vi "App - analyze RUS V6.vi"() -> ()   [LabVIEW 2018] (continued)
  in  "t.folder file path array":T26[](array[typedef])=[{"temperature"=241.719, "temperature str"="241.71900", "file path"=path "D:/Data/Ultrasound/LSCO/LSCO22__130814c/5_Cooling_2nd_try/September_2014/091614/241.71900K_500_2500_2.10000V_0.00000T_Sep16-2014__11-57-01_001_091614.bin", "last mod"=timestamp(3493727821 s since 1904-01-01), "file name str"="D:\\Data\\Ultrasound\\LSCO\\LSCO22__130814c\\5_Cooling_2nd_try\\September_2014\\091614\\241.71900K_500_2500_2.10000V_0.00000T_Sep16-2014__11-57-01_001_091614.bin", "mod time(min)"=58228797.016666666, "file format"=enum."binary", "power(V)"=2.1, "Magn Field(T) "=0.0}, {"temperature"=220.002, "temperature str"="220.00200", "file path"=path "D:/Data/Ultrasound/LSCO/LSCO22__130814c/5_Cooling_2nd_try/September_2014/091614/220.00200K_500_2500_2.10000V_0.00000T_Sep16-2014__12-18-19_001_091614.bin", "last mod"=timestamp(3493729099 s since 1904-01-01), "file name str"="D:\\Data\\Ultrasound\\LSCO\\LSCO22__130814c\\5_Cooling_2nd_try\\September_2014\\091614\\220.00200K_500_2500_2.10000V_0.00000T_Sep16-2014__12-18-19_001_091614.bin", "mod time(min)"=58228818.31666667, "file format"=enum."binary", "power(V)"=2.1, "Magn Field(T) "=0.0}, {"temperature"=219.999, "temperature str"="219.99900", "file path"=path "D:/Data/Ultrasound/LSCO/LSCO22__130814c/5_Cooling_2nd_try/September_2014/091614/219.99900K_500_2500_2.10000V_0.00000T_Sep16-2014__12-20-36_001_091614.bin", "last mod"=timestamp(3493729236 s since 1904-01-01), "file name str"="D:\\Data\\Ultrasound\\LSCO\\LSCO22__130814c\\5_Cooling_2nd_try\\September_2014\\091614\\219.99900K_500_2500_2.10000V_0.00000T_Sep16-2014__12-20-36_001_091614.bin", "mod time(min)"=58228820.6, "file format"=enum."binary", "power(V)"=2.1, "Magn Field(T) "=0.0}, {"temperature"=220.002, "temperature str"="220.00200", "file path"=path "D:/Data/Ultrasound/LSCO/LSCO22__130814c/5_Cooling_2nd_try/September_2014/091614/220.00200K_500_2500_2.10000V_0.00000T_Sep16-2014__12-21-56_001_091614.bin", "last mod"=timestamp(3493729316 s since 1904-01-01), "file name str"="D:\\Data\\Ultrasound\\LSCO\\LSCO22__130814c\\5_Cooling_2nd_try\\September_2014\\091614\\220.00200K_500_2500_2.10000V_0.00000T_Sep16-2014__12-21-56_001_091614.bin", "mod time(min)"=58228821.93333333, "file format"=enum."binary", "power(V)"=2.1, "Magn Field(T) "=0.0}, {"temperature"=221.376, "temperature str"="221.37600", "file path"=path "D:/Data/Ultrasound/LSCO/LSCO22__130814c/5_Cooling_2nd_try/September_2014/091614/221.37600K_500_2500_2.10000V_0.00000T_Sep16-2014__12-23-15_001_091614.bin", "last mod"=timestamp(3493729395 s since 1904-01-01), "file name str"="D:\\Data\\Ultrasound\\LSCO\\LSCO22__130814c\\5_Cooling_2nd_try\\September_2014\\091614\\221.37600K_500_2500_2.10000V_0.00000T_Sep16-2014__12-23-15_001_091614.bin", "mod time(min)"=58228823.25, "file format"=enum."binary", "power(V)"=2.1, "Magn Field(T) "=0.0}, {"temperature"=220.736, "temperature str"="220.73600", "file path"=path "D:/Data/Ultrasound/LSCO/LSCO22__130814c/5_Cooling_2nd_try/September_2014/091614/220.73600K_500_2500_2.10000V_0.00000T_Sep16-2014__12-24-35_001_091614.bin", "last mod"=timestamp(3493729475 s since 1904-01-01), "file name str"="D:\\Data\\Ultrasound\\LSCO\\LSCO22__130814c\\5_Cooling_2nd_try\\September_2014\\091614\\220.73600K_500_2500_2.10000V_0.00000T_Sep16-2014__12-24-35_001_091614.bin", "mod time(min)"=58228824.583333336, "file format"=enum."binary", "power(V)"=2.1, "Magn Field(T) "=0.0}, {"temperature"=220.112, "temperature str"="220.11200", "file path"=path "D:/Data/Ultrasound/LSCO/LSCO22__130814c/5_Cooling_2nd_try/September_2014/091614/220.11200K_500_2500_2.10000V_0.00000T_Sep16-2014__12-25-54_001_091614.bin", "last mod"=timestamp(3493729554 s since 1904-01-01), "file name str"="D:\\Data\\Ultrasound\\LSCO\\LSCO22__130814c\\5_Cooling_2nd_try\\September_2014\\091614\\220.11200K_500_2500_2.10000V_0.00000T_Sep16-2014__12-25-54_001_091614.bin", "mod time(min)"=58228825.9, "file format"=enum."binary", "power(V)"=2.1, "Magn Field(T) "=0.0}, {"temperature"=219.885, "temperature str"="219.88500", "file path"=path "D:/Data/Ultrasound/LSCO/LSCO22__130814c/5_Cooling_2nd_try/September_2014/091614/219.88500K_500_2500_2.10000V_0.00000T_Sep16-2014__12-27-13_001_091614.bin", "last mod"=timestamp(3493729633 s since 1904-01-01), "file name str"="D:\\Data\\Ultrasound\\LSCO\\LSCO22__130814c\\5_Cooling_2nd_try\\September_2014\\091614\\219.88500K_500_2500_2.10000V_0.00000T_Sep16-2014__12-27-13_001_091614.bin", "mod time(min)"=58228827.21666667, "file format"=enum."binary", "power(V)"=2.1, "Magn Field(T) "=0.0}, {"temperature"=219.907, "temperature str"="219.90700", "file path"=path "D:/Data/Ultrasound/LSCO/LSCO22__130814c/5_Cooling_2nd_try/September_2014/091614/219.90700K_500_2500_2.10000V_0.00000T_Sep16-2014__12-28-33_001_091614.bin", "last mod"=timestamp(3493729713 s since 1904-01-01), "file name str"="D:\\Data\\Ultrasound\\LSCO\\LSCO22__130814c\\5_Cooling_2nd_try\\September_2014\\091614\\219.90700K_500_2500_2.10000V_0.00000T_Sep16-2014__12-28-33_001_091614.bin", "mod time(min)"=58228828.55, "file format"=enum."binary", "power(V)"=2.1, "Magn Field(T) "=0.0}, {"temperature"=220.061, "temperature str"="220.06100", "file path"=path "D:/Data/Ultrasound/LSCO/LSCO22__130814c/5_Cooling_2nd_try/September_2014/091614/220.06100K_500_2500_2.10000V_0.00000T_Sep16-2014__12-29-52_001_091614.bin", "last mod"=timestamp(3493729792 s since 1904-01-01), "file name str"="D:\\Data\\Ultrasound\\LSCO\\LSCO22__130814c\\5_Cooling_2nd_try\\September_2014\\091614\\220.06100K_500_2500_2.10000V_0.00000T_Sep16-2014__12-29-52_001_091614.bin", "mod time(min)"=58228829.86666667, "file format"=enum."binary", "power(V)"=2.1, "Magn Field(T) "=0.0}, {"temperature"=220.167, "temperature str"="220.16700", "file path"=path "D:/Data/Ultrasound/LSCO/LSCO22__130814c/5_Cooling_2nd_try/September_2014/091614/220.16700K_500_2500_2.10000V_0.00000T_Sep16-2014__12-31-11_001_091614.bin", "last mod"=timestamp(3493729871 s since 1904-01-01), "file name str"="D:\\Data\\Ultrasound\\LSCO\\LSCO22__130814c\\5_Cooling_2nd_try\\September_2014\\091614\\220.16700K_500_2500_2.10000V_0.00000T_Sep16-2014__12-31-11_001_091614.bin", "mod time(min)"=58228831.18333333, "file format"=enum."binary", "power(V)"=2.1, "Magn Field(T) "=0.0}, {"temperature"=220.232, "temperature str"="220.23200", "file path"=path "D:/Data/Ultrasound/LSCO/LSCO22__130814c/5_Cooling_2nd_try/September_2014/091614/220.23200K_500_2500_2.10000V_0.00000T_Sep16-2014__12-32-31_001_091614.bin", "last mod"=timestamp(3493729951 s since 1904-01-01), "file name str"="D:\\Data\\Ultrasound\\LSCO\\LSCO22__130814c\\5_Cooling_2nd_try\\September_2014\\091614\\220.23200K_500_2500_2.10000V_0.00000T_Sep16-2014__12-32-31_001_091614.bin", "mod time(min)"=58228832.516666666, "file format"=enum."binary", "power(V)"=2.1, "Magn Field(T) "=0.0}, {"temperature"=220.32, "temperature str"="220.32000", "file path"=path "D:/Data/Ultrasound/LSCO/LSCO22__130814c/5_Cooling_2nd_try/September_2014/091614/220.32000K_500_2500_2.10000V_0.00000T_Sep16-2014__12-33-50_001_091614.bin", "last mod"=timestamp(3493730030 s since 1904-01-01), "file name str"="D:\\Data\\Ultrasound\\LSCO\\LSCO22__130814c\\5_Cooling_2nd_try\\September_2014\\091614\\220.32000K_500_2500_2.10000V_0.00000T_Sep16-2014__12-33-50_001_091614.bin", "mod time(min)"=58228833.833333336, "file format"=enum."binary", "power(V)"=2.1, "Magn Field(T) "=0.0}, {"temperature"=220.447, "temperature str"="220.44700", "file path"=path "D:/Data/Ultrasound/LSCO/LSCO22__130814c/5_Cooling_2nd_try/September_2014/091614/220.44700K_500_2500_2.10000V_0.00000T_Sep16-2014__12-35-10_001_091614.bin", "last mod"=timestamp(3493730110 s since 1904-01-01), "file name str"="D:\\Data\\Ultrasound\\LSCO\\LSCO22__130814c\\5_Cooling_2nd_try\\September_2014\\091614\\220.44700K_500_2500_2.10000V_0.00000T_Sep16-2014__12-35-10_001_091614.bin", "mod time(min)"=58228835.166666664, "file format"=enum."binary", "power(V)"=2.1, "Magn Field(T) "=0.0}, {"temperature"=220.033, "temperature str"="220.03300", "file path"=path "D:/Data/Ultrasound/LSCO/LSCO22__130814c/5_Cooling_2nd_try/September_2014/091614/220.03300K_500_2500_2.10000V_0.00000T_Sep16-2014__12-36-29_001_091614.bin", "last mod"=timestamp(3493730189 s since 1904-01-01), "file name str"="D:\\Data\\Ultrasound\\LSCO\\LSCO22__130814c\\5_Cooling_2nd_try\\September_2014\\091614\\220.03300K_500_2500_2.10000V_0.00000T_Sep16-2014__12-36-29_001_091614.bin", "mod time(min)"=58228836.483333334, "file format"=enum."binary", "power(V)"=2.1, "Magn Field(T) "=0.0}, {"temperature"=219.225, "temperature str"="219.22500", "file path"=path "D:/Data/Ultrasound/LSCO/LSCO22__130814c/5_Cooling_2nd_try/September_2014/091614/219.22500K_500_2500_2.10000V_0.00000T_Sep16-2014__12-37-48_001_091614.bin", "last mod"=timestamp(3493730268 s since 1904-01-01), "file name str"="D:\\Data\\Ultrasound\\LSCO\\LSCO22__130814c\\5_Cooling_2nd_try\\September_2014\\091614\\219.22500K_500_2500_2.10000V_0.00000T_Sep16-2014__12-37-48_001_091614.bin", "mod time(min)"=58228837.8, "file format"=enum."binary", "power(V)"=2.1, "Magn Field(T) "=0.0}, {"temperature"=219.76, "temperature str"="219.76000", "file path"=path "D:/Data/Ultrasound/LSCO/LSCO22__130814c/5_Cooling_2nd_try/September_2014/091614/219.76000K_500_2500_2.10000V_0.00000T_Sep16-2014__12-39-08_001_091614.bin", "last mod"=timestamp(3493730348 s since 1904-01-01), "file name str"="D:\\Data\\Ultrasound\\LSCO\\LSCO22__130814c\\5_Cooling_2nd_try\\September_2014\\091614\\219.76000K_500_2500_2.10000V_0.00000T_Sep16-2014__12-39-08_001_091614.bin", "mod time(min)"=58228839.13333333, "file format"=enum."binary", "power(V)"=2.1, "Magn Field(T) "=0.0}, {"temperature"=220.195, "temperature str"="220.19500", "file path"=path "D:/Data/Ultrasound/LSCO/LSCO22__130814c/5_Cooling_2nd_try/September_2014/091614/220.19500K_500_2500_2.10000V_0.00000T_Sep16-2014__12-40-27_001_091614.bin", "last mod"=timestamp(3493730427 s since 1904-01-01), "file name str"="D:\\Data\\Ultrasound\\LSCO\\LSCO22__130814c\\5_Cooling_2nd_try\\September_2014\\091614\\220.19500K_500_2500_2.10000V_0.00000T_Sep16-2014__12-40-27_001_091614.bin", "mod time(min)"=58228840.45, "file format"=enum."binary", "power(V)"=2.1, "Magn Field(T) "=0.0}, {"temperature"=219.549, "temperature str"="219.54900", "file path"=path "D:/Data/Ultrasound/LSCO/LSCO22__130814c/5_Cooling_2nd_try/September_2014/091614/219.54900K_500_2500_2.10000V_0.00000T_Sep16-2014__12-41-46_001_091614.bin", "last mod"=timestamp(3493730506 s since 1904-01-01), "file name str"="D:\\Data\\Ultrasound\\LSCO\\LSCO22__130814c\\5_Cooling_2nd_try\\September_2014\\091614\\219.54900K_500_2500_2.10000V_0.00000T_Sep16-2014__12-41-46_001_091614.bin", "mod time(min)"=58228841.766666666, "file format"=enum."binary", "power(V)"=2.1, "Magn Field(T) "=0.0}, {"temperature"=219.085, "temperature str"="219.08500", "file path"=path "D:/Data/Ultrasound/LSCO/LSCO22__130814c/5_Cooling_2nd_try/September_2014/091614/219.08500K_500_2500_2.10000V_0.00000T_Sep16-2014__12-43-06_001_091614.bin", "last mod"=timestamp(3493730586 s since 1904-01-01), "file name str"="D:\\Data\\Ultrasound\\LSCO\\LSCO22__130814c\\5_Cooling_2nd_try\\September_2014\\091614\\219.08500K_500_2500_2.10000V_0.00000T_Sep16-2014__12-43-06_001_091614.bin", "mod time(min)"=58228843.1, "file format"=enum."binary", "power(V)"=2.1, "Magn Field(T) "=0.0}, {"temperature"=219.006, "temperature str"="219.00600", "file path"=path "D:/Data/Ultrasound/LSCO/LSCO22__130814c/5_Cooling_2nd_try/September_2014/091614/219.00600K_500_2500_2.10000V_0.00000T_Sep16-2014__12-44-25_001_091614.bin", "last mod"=timestamp(3493730665 s since 1904-01-01), "file name str"="D:\\Data\\Ultrasound\\LSCO\\LSCO22__130814c\\5_Cooling_2nd_try\\September_2014\\091614\\219.00600K_500_2500_2.10000V_0.00000T_Sep16-2014__12-44-25_001_091614.bin", "mod time(min)"=58228844.416666664, "file format"=enum."binary", "power(V)"=2.1, "Magn Field(T) "=0.0}, {"temperature"=218.791, "temperature str"="218.79100", "file path"=path "D:/Data/Ultrasound/LSCO/LSCO22__130814c/5_Cooling_2nd_try/September_2014/091614/218.79100K_500_2500_2.10000V_0.00000T_Sep16-2014__12-45-45_001_091614.bin", "last mod"=timestamp(3493730745 s since 1904-01-01), "file name str"="D:\\Data\\Ultrasound\\LSCO\\LSCO22__130814c\\5_Cooling_2nd_try\\September_2014\\091614\\218.79100K_500_2500_2.10000V_0.00000T_Sep16-2014__12-45-45_001_091614.bin", "mod time(min)"=58228845.75, "file format"=enum."binary", "power(V)"=2.1, "Magn Field(T) "=0.0}, {"temperature"=218.445, "temperature str"="218.44500", "file path"=path "D:/Data/Ultrasound/LSCO/LSCO22__130814c/5_Cooling_2nd_try/September_2014/091614/218.44500K_500_2500_2.10000V_0.00000T_Sep16-2014__12-47-04_001_091614.bin", "last mod"=timestamp(3493730824 s since 1904-01-01), "file name str"="D:\\Data\\Ultrasound\\LSCO\\LSCO22__130814c\\5_Cooling_2nd_try\\September_2014\\091614\\218.44500K_500_2500_2.10000V_0.00000T_Sep16-2014__12-47-04_001_091614.bin", "mod time(min)"=58228847.06666667, "file format"=enum."binary", "power(V)"=2.1, "Magn Field(T) "=0.0}, {"temperature"=218.177, "temperature str"="218.17700", "file path"=path "D:/Data/Ultrasound/LSCO/LSCO22__130814c/5_Cooling_2nd_try/September_2014/091614/218.17700K_500_2500_2.10000V_0.00000T_Sep16-2014__12-48-23_001_091614.bin", "last mod"=timestamp(3493730903 s since 1904-01-01), "file name str"="D:\\Data\\Ultrasound\\LSCO\\LSCO22__130814c\\5_Cooling_2nd_try\\September_2014\\091614\\218.17700K_500_2500_2.10000V_0.00000T_Sep16-2014__12-48-23_001_091614.bin", "mod time(min)"=58228848.38333333, "file format"=enum."binary", "power(V)"=2.1, "Magn Field(T) "=0.0}, {"temperature"=217.946, "temperature str"="217.94600", "file path"=path "D:/Data/Ultrasound/LSCO/LSCO22__130814c/5_Cooling_2nd_try/September_2014/091614/217.94600K_500_2500_2.10000V_0.00000T_Sep16-2014__12-49-43_001_091614.bin", "last mod"=timestamp(3493730983 s since 1904-01-01), "file name str"="D:\\Data\\Ultrasound\\LSCO\\LSCO22__130814c\\5_Cooling_2nd_try\\September_2014\\091614\\217.94600K_500_2500_2.10000V_0.00000T_Sep16-2014__12-49-43_001_091614.bin", "mod time(min)"=58228849.71666667, "file format"=enum."binary", "power(V)"=2.1, "Magn Field(T) "=0.0}, {"temperature"=217.689, "temperature str"="217.68900", "file path"=path "D:/Data/Ultrasound/LSCO/LSCO22__130814c/5_Cooling_2nd_try/September_2014/091614/217.68900K_500_2500_2.10000V_0.00000T_Sep16-2014__12-51-02_001_091614.bin", "last mod"=timestamp(3493731062 s since 1904-01-01), "file name str"="D:\\Data\\Ultrasound\\LSCO\\LSCO22__130814c\\5_Cooling_2nd_try\\September_2014\\091614\\217.68900K_500_2500_2.10000V_0.00000T_Sep16-2014__12-51-02_001_091614.bin", "mod time(min)"=58228851.03333333, "file format"=enum."binary", "power(V)"=2.1, "Magn Field(T) "=0.0}, {"temperature"=217.41, "temperature str"="217.41000", "file path"=path "D:/Data/Ultrasound/LSCO/LSCO22__130814c/5_Cooling_2nd_try/September_2014/091614/217.41000K_500_2500_2.10000V_0.00000T_Sep16-2014__12-52-21_001_091614.bin", "last mod"=timestamp(3493731141 s since 1904-01-01), "file name str"="D:\\Data\\Ultrasound\\LSCO\\LSCO22__130814c\\5_Cooling_2nd_try\\September_2014\\091614\\217.41000K_500_2500_2.10000V_0.00000T_Sep16-2014__12-52-21_001_091614.bin", "mod time(min)"=58228852.35, "file format"=enum."binary", "power(V)"=2.1, "Magn Field(T) "=0.0}, {"temperature"=217.145, "temperature str"="217.14500", "file path"=path "D:/Data/Ultrasound/LSCO/LSCO22__130814c/5_Cooling_2nd_try/September_2014/091614/217.14500K_500_2500_2.10000V_0.00000T_Sep16-2014__12-53-41_001_091614.bin", "last mod"=timestamp(3493731221 s since 1904-01-01), "file name str"="D:\\Data\\Ultrasound\\LSCO\\LSCO22__130814c\\5_Cooling_2nd_try\\September_2014\\091614\\217.14500K_500_2500_2.10000V_0.00000T_Sep16-2014__12-53-41_001_091614.bin", "mod time(min)"=58228853.68333333, "file format"=enum."binary", "power(V)"=2.1, "Magn Field(T) "=0.0}, {"temperature"=216.895, "temperature str"="216.89500", "file path"=path "D:/Data/Ultrasound/LSCO/LSCO22__130814c/5_Cooling_2nd_try/September_2014/091614/216.89500K_500_2500_2.10000V_0.00000T_Sep16-2014__12-55-00_001_091614.bin", "last mod"=timestamp(3493731300 s since 1904-01-01), "file name str"="D:\\Data\\Ultrasound\\LSCO\\LSCO22__130814c\\5_Cooling_2nd_try\\September_2014\\091614\\216.89500K_500_2500_2.10000V_0.00000T_Sep16-2014__12-55-00_001_091614.bin", "mod time(min)"=58228855.0, "file format"=enum."binary", "power(V)"=2.1, "Magn Field(T) "=0.0}, {"temperature"=216.629, "temperature str"="216.62900", "file path"=path "D:/Data/Ultrasound/LSCO/LSCO22__130814c/5_Cooling_2nd_try/September_2014/091614/216.62900K_500_2500_2.10000V_0.00000T_Sep16-2014__12-56-20_001_091614.bin", "last mod"=timestamp(3493731380 s since 1904-01-01), "file name str"="D:\\Data\\Ultrasound\\LSCO\\LSCO22__130814c\\5_Cooling_2nd_try\\September_2014\\091614\\216.62900K_500_2500_2.10000V_0.00000T_Sep16-2014__12-56-20_001_091614.bin", "mod time(min)"=58228856.333333336, "file format"=enum."binary", "power(V)"=2.1, "Magn Field(T) "=0.0}, {"temperature"=216.359, "temperature str"="216.35900", "file path"=path "D:/Data/Ultrasound/LSCO/LSCO22__130814c/5_Cooling_2nd_try/September_2014/091614/216.35900K_500_2500_2.10000V_0.00000T_Sep16-2014__12-57-39_001_091614.bin", "last mod"=timestamp(3493731459 s since 1904-01-01), "file name str"="D:\\Data\\Ultrasound\\LSCO\\LSCO22__130814c\\5_Cooling_2nd_try\\September_2014\\091614\\216.35900K_500_2500_2.10000V_0.00000T_Sep16-2014__12-57-39_001_091614.bin", "mod time(min)"=58228857.65, "file format"=enum."binary", "power(V)"=2.1, "Magn Field(T) "=0.0}, {"temperature"=216.106, "temperature str"="216.10600", "file path"=path "D:/Data/Ultrasound/LSCO/LSCO22__130814c/5_Cooling_2nd_try/September_2014/091614/216.10600K_500_2500_2.10000V_0.00000T_Sep16-2014__12-58-58_001_091614.bin", "last mod"=timestamp(3493731538 s since 1904-01-01), "file name str"="D:\\Data\\Ultrasound\\LSCO\\LSCO22__130814c\\5_Cooling_2nd_try\\September_2014\\091614\\216.10600K_500_2500_2.10000V_0.00000T_Sep16-2014__12-58-58_001_091614.bin", "mod time(min)"=58228858.96666667, "file format"=enum."binary", "power(V)"=2.1, "Magn Field(T) "=0.0}, {"temperature"=215.839, "temperature str"="215.83900", "file path"=path "D:/Data/Ultrasound/LSCO/LSCO22__130814c/5_Cooling_2nd_try/September_2014/091614/215.83900K_500_2500_2.10000V_0.00000T_Sep16-2014__13-00-18_001_091614.bin", "last mod"=timestamp(3493731618 s since 1904-01-01), "file name str"="D:\\Data\\Ultrasound\\LSCO\\LSCO22__130814c\\5_Cooling_2nd_try\\September_2014\\091614\\215.83900K_500_2500_2.10000V_0.00000T_Sep16-2014__13-00-18_001_091614.bin", "mod time(min)"=58228860.3, "file format"=enum."binary", "power(V)"=2.1, "Magn Field(T) "=0.0}, {"temperature"=215.585, "temperature str"="215.58500", "file path"=path "D:/Data/Ultrasound/LSCO/LSCO22__130814c/5_Cooling_2nd_try/September_2014/091614/215.58500K_500_2500_2.10000V_0.00000T_Sep16-2014__13-01-37_001_091614.bin", "last mod"=timestamp(3493731697 s since 1904-01-01), "file name str"="D:\\Data\\Ultrasound\\LSCO\\LSCO22__130814c\\5_Cooling_2nd_try\\September_2014\\091614\\215.58500K_500_2500_2.10000V_0.00000T_Sep16-2014__13-01-37_001_091614.bin", "mod time(min)"=58228861.61666667, "file format"=enum."binary", "power(V)"=2.1, "Magn Field(T) "=0.0}, {"temperature"=215.319, "temperature str"="215.31900", "file path"=path "D:/Data/Ultrasound/LSCO/LSCO22__130814c/5_Cooling_2nd_try/September_2014/091614/215.31900K_500_2500_2.10000V_0.00000T_Sep16-2014__13-02-56_001_091614.bin", "last mod"=timestamp(3493731776 s since 1904-01-01), "file name str"="D:\\Data\\Ultrasound\\LSCO\\LSCO22__130814c\\5_Cooling_2nd_try\\September_2014\\091614\\215.31900K_500_2500_2.10000V_0.00000T_Sep16-2014__13-02-56_001_091614.bin", "mod time(min)"=58228862.93333333, "file format"=enum."binary", "power(V)"=2.1, "Magn Field(T) "=0.0}, {"temperature"=215.053, "temperature str"="215.05300", "file path"=path "D:/Data/Ultrasound/LSCO/LSCO22__130814c/5_Cooling_2nd_try/September_2014/091614/215.05300K_500_2500_2.10000V_0.00000T_Sep16-2014__13-04-16_001_091614.bin", "last mod"=timestamp(3493731856 s since 1904-01-01), "file name str"="D:\\Data\\Ultrasound\\LSCO\\LSCO22__130814c\\5_Cooling_2nd_try\\September_2014\\091614\\215.05300K_500_2500_2.10000V_0.00000T_Sep16-2014__13-04-16_001_091614.bin", "mod time(min)"=58228864.266666666, "file format"=enum."binary", "power(V)"=2.1, "Magn Field(T) "=0.0}, {"temperature"=214.797, "temperature str"="214.79700", "file path"=path "D:/Data/Ultrasound/LSCO/LSCO22__130814c/5_Cooling_2nd_try/September_2014/091614/214.79700K_500_2500_2.10000V_0.00000T_Sep16-2014__13-05-35_001_091614.bin", "last mod"=timestamp(3493731935 s since 1904-01-01), "file name str"="D:\\Data\\Ultrasound\\LSCO\\LSCO22__130814c\\5_Cooling_2nd_try\\September_2014\\091614\\214.79700K_500_2500_2.10000V_0.00000T_Sep16-2014__13-05-35_001_091614.bin", "mod time(min)"=58228865.583333336, "file format"=enum."binary", "power(V)"=2.1, "Magn Field(T) "=0.0}, {"temperature"=214.531, "temperature str"="214.53100", "file path"=path "D:/Data/Ultrasound/LSCO/LSCO22__130814c/5_Cooling_2nd_try/September_2014/091614/214.53100K_500_2500_2.10000V_0.00000T_Sep16-2014__13-06-55_001_091614.bin", "last mod"=timestamp(3493732015 s since 1904-01-01), "file name str"="D:\\Data\\Ultrasound\\LSCO\\LSCO22__130814c\\5_Cooling_2nd_try\\September_2014\\091614\\214.53100K_500_2500_2.10000V_0.00000T_Sep16-2014__13-06-55_001_091614.bin", "mod time(min)"=58228866.916666664, "file format"=enum."binary", "power(V)"=2.1, "Magn Field(T) "=0.0}, {"temperature"=214.276, "temperature str"="214.27600", "file path"=path "D:/Data/Ultrasound/LSCO/LSCO22__130814c/5_Cooling_2nd_try/September_2014/091614/214.27600K_500_2500_2.10000V_0.00000T_Sep16-2014__13-08-14_001_091614.bin", "last mod"=timestamp(3493732094 s since 1904-01-01), "file name str"="D:\\Data\\Ultrasound\\LSCO\\LSCO22__130814c\\5_Cooling_2nd_try\\September_2014\\091614\\214.27600K_500_2500_2.10000V_0.00000T_Sep16-2014__13-08-14_001_091614.bin", "mod time(min)"=58228868.233333334, "file format"=enum."binary", "power(V)"=2.1, "Magn Field(T) "=0.0}, {"temperature"=214.01, "temperature str"="214.01000", "file path"=path "D:/Data/Ultrasound/LSCO/LSCO22__130814c/5_Cooling_2nd_try/September_2014/091614/214.01000K_500_2500_2.10000V_0.00000T_Sep16-2014__13-09-33_001_091614.bin", "last mod"=timestamp(3493732173 s since 1904-01-01), "file name str"="D:\\Data\\Ultrasound\\LSCO\\LSCO22__130814c\\5_Cooling_2nd_try\\September_2014\\091614\\214.01000K_500_2500_2.10000V_0.00000T_Sep16-2014__13-09-33_001_091614.bin", "mod time(min)"=58228869.55, "file format"=enum."binary", "power(V)"=2.1, "Magn Field(T) "=0.0}, {"temperature"=213.745, "temperature str"="213.74500", "file path"=path "D:/Data/Ultrasound/LSCO/LSCO22__130814c/5_Cooling_2nd_try/September_2014/091614/213.74500K_500_2500_2.10000V_0.00000T_Sep16-2014__13-10-53_001_091614.bin", "last mod"=timestamp(3493732253 s since 1904-01-01), "file name str"="D:\\Data\\Ultrasound\\LSCO\\LSCO22__130814c\\5_Cooling_2nd_try\\September_2014\\091614\\213.74500K_500_2500_2.10000V_0.00000T_Sep16-2014__13-10-53_001_091614.bin", "mod time(min)"=58228870.88333333, "file format"=enum."binary", "power(V)"=2.1, "Magn Field(T) "=0.0}, {"temperature"=213.49, "temperature str"="213.49000", "file path"=path "D:/Data/Ultrasound/LSCO/LSCO22__130814c/5_Cooling_2nd_try/September_2014/091614/213.49000K_500_2500_2.10000V_0.00000T_Sep16-2014__13-12-12_001_091614.bin", "last mod"=timestamp(3493732332 s since 1904-01-01), "file name str"="D:\\Data\\Ultrasound\\LSCO\\LSCO22__130814c\\5_Cooling_2nd_try\\September_2014\\091614\\213.49000K_500_2500_2.10000V_0.00000T_Sep16-2014__13-12-12_001_091614.bin", "mod time(min)"=58228872.2, "file format"=enum."binary", "power(V)"=2.1, "Magn Field(T) "=0.0}, {"temperature"=213.225, "temperature str"="213.22500", "file path"=path "D:/Data/Ultrasound/LSCO/LSCO22__130814c/5_Cooling_2nd_try/September_2014/091614/213.22500K_500_2500_2.10000V_0.00000T_Sep16-2014__13-13-31_001_091614.bin", "last mod"=timestamp(3493732411 s since 1904-01-01), "file name str"="D:\\Data\\Ultrasound\\LSCO\\LSCO22__130814c\\5_Cooling_2nd_try\\September_2014\\091614\\213.22500K_500_2500_2.10000V_0.00000T_Sep16-2014__13-13-31_001_091614.bin", "mod time(min)"=58228873.516666666, "file format"=enum."binary", "power(V)"=2.1, "Magn Field(T) "=0.0}, {"temperature"=212.968, "temperature str"="212.96800", "file path"=path "D:/Data/Ultrasound/LSCO/LSCO22__130814c/5_Cooling_2nd_try/September_2014/091614/212.96800K_500_2500_2.10000V_0.00000T_Sep16-2014__13-14-51_001_091614.bin", "last mod"=timestamp(3493732491 s since 1904-01-01), "file name str"="D:\\Data\\Ultrasound\\LSCO\\LSCO22__130814c\\5_Cooling_2nd_try\\September_2014\\091614\\212.96800K_500_2500_2.10000V_0.00000T_Sep16-2014__13-14-51_001_091614.bin", "mod time(min)"=58228874.85, "file format"=enum."binary", "power(V)"=2.1, "Magn Field(T) "=0.0}, {"temperature"=212.699, "temperature str"="212.69900", "file path"=path "D:/Data/Ultrasound/LSCO/LSCO22__130814c/5_Cooling_2nd_try/September_2014/091614/212.69900K_500_2500_2.10000V_0.00000T_Sep16-2014__13-16-10_001_091614.bin", "last mod"=timestamp(3493732570 s since 1904-01-01), "file name str"="D:\\Data\\Ultrasound\\LSCO\\LSCO22__130814c\\5_Cooling_2nd_try\\September_2014\\091614\\212.69900K_500_2500_2.10000V_0.00000T_Sep16-2014__13-16-10_001_091614.bin", "mod time(min)"=58228876.166666664, "file format"=enum."binary", "power(V)"=2.1, "Magn Field(T) "=0.0}, {"temperature"=212.433, "temperature str"="212.43300", "file path"=path "D:/Data/Ultrasound/LSCO/LSCO22__130814c/5_Cooling_2nd_try/September_2014/091614/212.43300K_500_2500_2.10000V_0.00000T_Sep16-2014__13-17-30_001_091614.bin", "last mod"=timestamp(3493732650 s since 1904-01-01), "file name str"="D:\\Data\\Ultrasound\\LSCO\\LSCO22__130814c\\5_Cooling_2nd_try\\September_2014\\091614\\212.43300K_500_2500_2.10000V_0.00000T_Sep16-2014__13-17-30_001_091614.bin", "mod time(min)"=58228877.5, "file format"=enum."binary", "power(V)"=2.1, "Magn Field(T) "=0.0}, {"temperature"=212.177, "temperature str"="212.17700", "file path"=path "D:/Data/Ultrasound/LSCO/LSCO22__130814c/5_Cooling_2nd_try/September_2014/091614/212.17700K_500_2500_2.10000V_0.00000T_Sep16-2014__13-18-49_001_091614.bin", "last mod"=timestamp(3493732729 s since 1904-01-01), "file name str"="D:\\Data\\Ultrasound\\LSCO\\LSCO22__130814c\\5_Cooling_2nd_try\\September_2014\\091614\\212.17700K_500_2500_2.10000V_0.00000T_Sep16-2014__13-18-49_001_091614.bin", "mod time(min)"=58228878.81666667, "file format"=enum."binary", "power(V)"=2.1, "Magn Field(T) "=0.0}, {"temperature"=211.909, "temperature str"="211.90900", "file path"=path "D:/Data/Ultrasound/LSCO/LSCO22__130814c/5_Cooling_2nd_try/September_2014/091614/211.90900K_500_2500_2.10000V_0.00000T_Sep16-2014__13-20-08_001_091614.bin", "last mod"=timestamp(3493732808 s since 1904-01-01), "file name str"="D:\\Data\\Ultrasound\\LSCO\\LSCO22__130814c\\5_Cooling_2nd_try\\September_2014\\091614\\211.90900K_500_2500_2.10000V_0.00000T_Sep16-2014__13-20-08_001_091614.bin", "mod time(min)"=58228880.13333333, "file format"=enum."binary", "power(V)"=2.1, "Magn Field(T) "=0.0}, {"temperature"=211.653, "temperature str"="211.65300", "file path"=path "D:/Data/Ultrasound/LSCO/LSCO22__130814c/5_Cooling_2nd_try/September_2014/091614/211.65300K_500_2500_2.10000V_0.00000T_Sep16-2014__13-21-28_001_091614.bin", "last mod"=timestamp(3493732888 s since 1904-01-01), "file name str"="D:\\Data\\Ultrasound\\LSCO\\LSCO22__130814c\\5_Cooling_2nd_try\\September_2014\\091614\\211.65300K_500_2500_2.10000V_0.00000T_Sep16-2014__13-21-28_001_091614.bin", "mod time(min)"=58228881.46666667, "file format"=enum."binary", "power(V)"=2.1, "Magn Field(T) "=0.0}, {"temperature"=211.386, "temperature str"="211.38600", "file path"=path "D:/Data/Ultrasound/LSCO/LSCO22__130814c/5_Cooling_2nd_try/September_2014/091614/211.38600K_500_2500_2.10000V_0.00000T_Sep16-2014__13-22-47_001_091614.bin", "last mod"=timestamp(3493732967 s since 1904-01-01), "file name str"="D:\\Data\\Ultrasound\\LSCO\\LSCO22__130814c\\5_Cooling_2nd_try\\September_2014\\091614\\211.38600K_500_2500_2.10000V_0.00000T_Sep16-2014__13-22-47_001_091614.bin", "mod time(min)"=58228882.78333333, "file format"=enum."binary", "power(V)"=2.1, "Magn Field(T) "=0.0}, {"temperature"=211.119, "temperature str"="211.11900", "file path"=path "D:/Data/Ultrasound/LSCO/LSCO22__130814c/5_Cooling_2nd_try/September_2014/091614/211.11900K_500_2500_2.10000V_0.00000T_Sep16-2014__13-24-06_001_091614.bin", "last mod"=timestamp(3493733046 s since 1904-01-01), "file name str"="D:\\Data\\Ultrasound\\LSCO\\LSCO22__130814c\\5_Cooling_2nd_try\\September_2014\\091614\\211.11900K_500_2500_2.10000V_0.00000T_Sep16-2014__13-24-06_001_091614.bin", "mod time(min)"=58228884.1, "file format"=enum."binary", "power(V)"=2.1, "Magn Field(T) "=0.0}, {"temperature"=210.861, "temperature str"="210.86100", "file path"=path "D:/Data/Ultrasound/LSCO/LSCO22__130814c/5_Cooling_2nd_try/September_2014/091614/210.86100K_500_2500_2.10000V_0.00000T_Sep16-2014__13-25-26_001_091614.bin", "last mod"=timestamp(3493733126 s since 1904-01-01), "file name str"="D:\\Data\\Ultrasound\\LSCO\\LSCO22__130814c\\5_Cooling_2nd_try\\September_2014\\091614\\210.86100K_500_2500_2.10000V_0.00000T_Sep16-2014__13-25-26_001_091614.bin", "mod time(min)"=58228885.43333333, "file format"=enum."binary", "power(V)"=2.1, "Magn Field(T) "=0.0}, {"temperature"=210.594, "temperature str"="210.59400", "file path"=path "D:/Data/Ultrasound/LSCO/LSCO22__130814c/5_Cooling_2nd_try/September_2014/091614/210.59400K_500_2500_2.10000V_0.00000T_Sep16-2014__13-26-45_001_091614.bin", "last mod"=timestamp(3493733205 s since 1904-01-01), "file name str"="D:\\Data\\Ultrasound\\LSCO\\LSCO22__130814c\\5_Cooling_2nd_try\\September_2014\\091614\\210.59400K_500_2500_2.10000V_0.00000T_Sep16-2014__13-26-45_001_091614.bin", "mod time(min)"=58228886.75, "file format"=enum."binary", "power(V)"=2.1, "Magn Field(T) "=0.0}, {"temperature"=210.336, "temperature str"="210.33600", "file path"=path "D:/Data/Ultrasound/LSCO/LSCO22__130814c/5_Cooling_2nd_try/September_2014/091614/210.33600K_500_2500_2.10000V_0.00000T_Sep16-2014__13-28-05_001_091614.bin", "last mod"=timestamp(3493733285 s since 1904-01-01), "file name str"="D:\\Data\\Ultrasound\\LSCO\\LSCO22__130814c\\5_Cooling_2nd_try\\September_2014\\091614\\210.33600K_500_2500_2.10000V_0.00000T_Sep16-2014__13-28-05_001_091614.bin", "mod time(min)"=58228888.083333336, "file format"=enum."binary", "power(V)"=2.1, "Magn Field(T) "=0.0}, {"temperature"=210.064, "temperature str"="210.06400", "file path"=path "D:/Data/Ultrasound/LSCO/LSCO22__130814c/5_Cooling_2nd_try/September_2014/091614/210.06400K_500_2500_2.10000V_0.00000T_Sep16-2014__13-29-24_001_091614.bin", "last mod"=timestamp(3493733364 s since 1904-01-01), "file name str"="D:\\Data\\Ultrasound\\LSCO\\LSCO22__130814c\\5_Cooling_2nd_try\\September_2014\\091614\\210.06400K_500_2500_2.10000V_0.00000T_Sep16-2014__13-29-24_001_091614.bin", "mod time(min)"=58228889.4, "file format"=enum."binary", "power(V)"=2.1, "Magn Field(T) "=0.0}, {"temperature"=209.8, "temperature str"="209.80000", "file path"=path "D:/Data/Ultrasound/LSCO/LSCO22__130814c/5_Cooling_2nd_try/September_2014/091614/209.80000K_500_2500_2.10000V_0.00000T_Sep16-2014__13-30-43_001_091614.bin", "last mod"=timestamp(3493733443 s since 1904-01-01), "file name str"="D:\\Data\\Ultrasound\\LSCO\\LSCO22__130814c\\5_Cooling_2nd_try\\September_2014\\091614\\209.80000K_500_2500_2.10000V_0.00000T_Sep16-2014__13-30-43_001_091614.bin", "mod time(min)"=58228890.71666667, "file format"=enum."binary", "power(V)"=2.1, "Magn Field(T) "=0.0}, {"temperature"=209.539, "temperature str"="209.53900", "file path"=path "D:/Data/Ultrasound/LSCO/LSCO22__130814c/5_Cooling_2nd_try/September_2014/091614/209.53900K_500_2500_2.10000V_0.00000T_Sep16-2014__13-32-03_001_091614.bin", "last mod"=timestamp(3493733523 s since 1904-01-01), "file name str"="D:\\Data\\Ultrasound\\LSCO\\LSCO22__130814c\\5_Cooling_2nd_try\\September_2014\\091614\\209.53900K_500_2500_2.10000V_0.00000T_Sep16-2014__13-32-03_001_091614.bin", "mod time(min)"=58228892.05, "file format"=enum."binary", "power(V)"=2.1, "Magn Field(T) "=0.0}, {"temperature"=209.267, "temperature str"="209.26700", "file path"=path "D:/Data/Ultrasound/LSCO/LSCO22__130814c/5_Cooling_2nd_try/September_2014/091614/209.26700K_500_2500_2.10000V_0.00000T_Sep16-2014__13-33-22_001_091614.bin", "last mod"=timestamp(3493733602 s since 1904-01-01), "file name str"="D:\\Data\\Ultrasound\\LSCO\\LSCO22__130814c\\5_Cooling_2nd_try\\September_2014\\091614\\209.26700K_500_2500_2.10000V_0.00000T_Sep16-2014__13-33-22_001_091614.bin", "mod time(min)"=58228893.36666667, "file format"=enum."binary", "power(V)"=2.1, "Magn Field(T) "=0.0}, {"temperature"=209.008, "temperature str"="209.00800", "file path"=path "D:/Data/Ultrasound/LSCO/LSCO22__130814c/5_Cooling_2nd_try/September_2014/091614/209.00800K_500_2500_2.10000V_0.00000T_Sep16-2014__13-34-42_001_091614.bin", "last mod"=timestamp(3493733682 s since 1904-01-01), "file name str"="D:\\Data\\Ultrasound\\LSCO\\LSCO22__130814c\\5_Cooling_2nd_try\\September_2014\\091614\\209.00800K_500_2500_2.10000V_0.00000T_Sep16-2014__13-34-42_001_091614.bin", "mod time(min)"=58228894.7, "file format"=enum."binary", "power(V)"=2.1, "Magn Field(T) "=0.0}, {"temperature"=208.737, "temperature str"="208.73700", "file path"=path "D:/Data/Ultrasound/LSCO/LSCO22__130814c/5_Cooling_2nd_try/September_2014/091614/208.73700K_500_2500_2.10000V_0.00000T_Sep16-2014__13-36-01_001_091614.bin", "last mod"=timestamp(3493733761 s since 1904-01-01), "file name str"="D:\\Data\\Ultrasound\\LSCO\\LSCO22__130814c\\5_Cooling_2nd_try\\September_2014\\091614\\208.73700K_500_2500_2.10000V_0.00000T_Sep16-2014__13-36-01_001_091614.bin", "mod time(min)"=58228896.016666666, "file format"=enum."binary", "power(V)"=2.1, "Magn Field(T) "=0.0}, {"temperature"=208.465, "temperature str"="208.46500", "file path"=path "D:/Data/Ultrasound/LSCO/LSCO22__130814c/5_Cooling_2nd_try/September_2014/091614/208.46500K_500_2500_2.10000V_0.00000T_Sep16-2014__13-37-20_001_091614.bin", "last mod"=timestamp(3493733840 s since 1904-01-01), "file name str"="D:\\Data\\Ultrasound\\LSCO\\LSCO22__130814c\\5_Cooling_2nd_try\\September_2014\\091614\\208.46500K_500_2500_2.10000V_0.00000T_Sep16-2014__13-37-20_001_091614.bin", "mod time(min)"=58228897.333333336, "file format"=enum."binary", "power(V)"=2.1, "Magn Field(T) "=0.0}, {"temperature"=208.205, "temperature str"="208.20500", "file path"=path "D:/Data/Ultrasound/LSCO/LSCO22__130814c/5_Cooling_2nd_try/September_2014/091614/208.20500K_500_2500_2.10000V_0.00000T_Sep16-2014__13-38-40_001_091614.bin", "last mod"=timestamp(3493733920 s since 1904-01-01), "file name str"="D:\\Data\\Ultrasound\\LSCO\\LSCO22__130814c\\5_Cooling_2nd_try\\September_2014\\091614\\208.20500K_500_2500_2.10000V_0.00000T_Sep16-2014__13-38-40_001_091614.bin", "mod time(min)"=58228898.666666664, "file format"=enum."binary", "power(V)"=2.1, "Magn Field(T) "=0.0}, {"temperature"=207.933, "temperature str"="207.93300", "file path"=path "D:/Data/Ultrasound/LSCO/LSCO22__130814c/5_Cooling_2nd_try/September_2014/091614/207.93300K_500_2500_2.10000V_0.00000T_Sep16-2014__13-39-59_001_091614.bin", "last mod"=timestamp(3493733999 s since 1904-01-01), "file name str"="D:\\Data\\Ultrasound\\LSCO\\LSCO22__130814c\\5_Cooling_2nd_try\\September_2014\\091614\\207.93300K_500_2500_2.10000V_0.00000T_Sep16-2014__13-39-59_001_091614.bin", "mod time(min)"=58228899.983333334, "file format"=enum."binary", "power(V)"=2.1, "Magn Field(T) "=0.0}, {"temperature"=207.67, "temperature str"="207.67000", "file path"=path "D:/Data/Ultrasound/LSCO/LSCO22__130814c/5_Cooling_2nd_try/September_2014/091614/207.67000K_500_2500_2.10000V_0.00000T_Sep16-2014__13-41-18_001_091614.bin", "last mod"=timestamp(3493734078 s since 1904-01-01), "file name str"="D:\\Data\\Ultrasound\\LSCO\\LSCO22__130814c\\5_Cooling_2nd_try\\September_2014\\091614\\207.67000K_500_2500_2.10000V_0.00000T_Sep16-2014__13-41-18_001_091614.bin", "mod time(min)"=58228901.3, "file format"=enum."binary", "power(V)"=2.1, "Magn Field(T) "=0.0}, {"temperature"=207.397, "temperature str"="207.39700", "file path"=path "D:/Data/Ultrasound/LSCO/LSCO22__130814c/5_Cooling_2nd_try/September_2014/091614/207.39700K_500_2500_2.10000V_0.00000T_Sep16-2014__13-42-38_001_091614.bin", "last mod"=timestamp(3493734158 s since 1904-01-01), "file name str"="D:\\Data\\Ultrasound\\LSCO\\LSCO22__130814c\\5_Cooling_2nd_try\\September_2014\\091614\\207.39700K_500_2500_2.10000V_0.00000T_Sep16-2014__13-42-38_001_091614.bin", "mod time(min)"=58228902.63333333, "file format"=enum."binary", "power(V)"=2.1, "Magn Field(T) "=0.0}, {"temperature"=207.121, "temperature str"="207.12100", "file path"=path "D:/Data/Ultrasound/LSCO/LSCO22__130814c/5_Cooling_2nd_try/September_2014/091614/207.12100K_500_2500_2.10000V_0.00000T_Sep16-2014__13-43-57_001_091614.bin", "last mod"=timestamp(3493734237 s since 1904-01-01), "file name str"="D:\\Data\\Ultrasound\\LSCO\\LSCO22__130814c\\5_Cooling_2nd_try\\September_2014\\091614\\207.12100K_500_2500_2.10000V_0.00000T_Sep16-2014__13-43-57_001_091614.bin", "mod time(min)"=58228903.95, "file format"=enum."binary", "power(V)"=2.1, "Magn Field(T) "=0.0}, {"temperature"=206.86, "temperature str"="206.86000", "file path"=path "D:/Data/Ultrasound/LSCO/LSCO22__130814c/5_Cooling_2nd_try/September_2014/091614/206.86000K_500_2500_2.10000V_0.00000T_Sep16-2014__13-45-17_001_091614.bin", "last mod"=timestamp(3493734317 s since 1904-01-01), "file name str"="D:\\Data\\Ultrasound\\LSCO\\LSCO22__130814c\\5_Cooling_2nd_try\\September_2014\\091614\\206.86000K_500_2500_2.10000V_0.00000T_Sep16-2014__13-45-17_001_091614.bin", "mod time(min)"=58228905.28333333, "file format"=enum."binary", "power(V)"=2.1, "Magn Field(T) "=0.0}, {"temperature"=206.586, "temperature str"="206.58600", "file path"=path "D:/Data/Ultrasound/LSCO/LSCO22__130814c/5_Cooling_2nd_try/September_2014/091614/206.58600K_500_2500_2.10000V_0.00000T_Sep16-2014__13-46-36_001_091614.bin", "last mod"=timestamp(3493734396 s since 1904-01-01), "file name str"="D:\\Data\\Ultrasound\\LSCO\\LSCO22__130814c\\5_Cooling_2nd_try\\September_2014\\091614\\206.58600K_500_2500_2.10000V_0.00000T_Sep16-2014__13-46-36_001_091614.bin", "mod time(min)"=58228906.6, "file format"=enum."binary", "power(V)"=2.1, "Magn Field(T) "=0.0}, {"temperature"=206.322, "temperature str"="206.32200", "file path"=path "D:/Data/Ultrasound/LSCO/LSCO22__130814c/5_Cooling_2nd_try/September_2014/091614/206.32200K_500_2500_2.10000V_0.00000T_Sep16-2014__13-47-55_001_091614.bin", "last mod"=timestamp(3493734475 s since 1904-01-01), "file name str"="D:\\Data\\Ultrasound\\LSCO\\LSCO22__130814c\\5_Cooling_2nd_try\\September_2014\\091614\\206.32200K_500_2500_2.10000V_0.00000T_Sep16-2014__13-47-55_001_091614.bin", "mod time(min)"=58228907.916666664, "file format"=enum."binary", "power(V)"=2.1, "Magn Field(T) "=0.0}, {"temperature"=206.047, "temperature str"="206.04700", "file path"=path "D:/Data/Ultrasound/LSCO/LSCO22__130814c/5_Cooling_2nd_try/September_2014/091614/206.04700K_500_2500_2.10000V_0.00000T_Sep16-2014__13-49-15_001_091614.bin", "last mod"=timestamp(3493734555 s since 1904-01-01), "file name str"="D:\\Data\\Ultrasound\\LSCO\\LSCO22__130814c\\5_Cooling_2nd_try\\September_2014\\091614\\206.04700K_500_2500_2.10000V_0.00000T_Sep16-2014__13-49-15_001_091614.bin", "mod time(min)"=58228909.25, "file format"=enum."binary", "power(V)"=2.1, "Magn Field(T) "=0.0}, {"temperature"=205.772, "temperature str"="205.77200", "file path"=path "D:/Data/Ultrasound/LSCO/LSCO22__130814c/5_Cooling_2nd_try/September_2014/091614/205.77200K_500_2500_2.10000V_0.00000T_Sep16-2014__13-50-34_001_091614.bin", "last mod"=timestamp(3493734634 s since 1904-01-01), "file name str"="D:\\Data\\Ultrasound\\LSCO\\LSCO22__130814c\\5_Cooling_2nd_try\\September_2014\\091614\\205.77200K_500_2500_2.10000V_0.00000T_Sep16-2014__13-50-34_001_091614.bin", "mod time(min)"=58228910.56666667, "file format"=enum."binary", "power(V)"=2.1, "Magn 
